vi "DeleteUser.vi"(3 "error in (no error)":errorcluster, 4 "User_Name":string, 5 "ID":string) -> (0 "error out":errorcluster)   [LabVIEW 2020]
uses:
  <vilib>/Utility/error.llb/DialogType.ctl
  Global1.vi
  <vilib>/addons/database/Connection.llb/DB Tools Open Connec (String).vi
  <vilib>/addons/database/Connection.llb/Conn Execute.vi
  <vilib>/addons/database/Recordset.llb/Rec Destroy - Connection.vi
  <vilib>/addons/database/NI_Database_API.lvlib
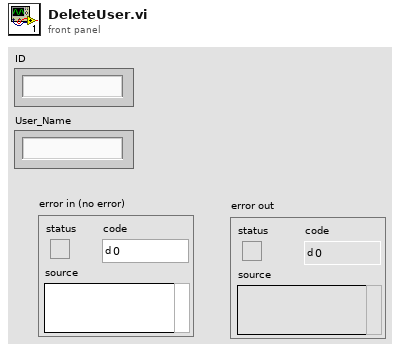
[diagram p1: front panel]
types:
  T1 = typedef "DialogType.ctl" = u16
  T2 = typedef "NI_Database_API.lvlib/Conn ObjectReference.ctl" = refnum<k1>
  T3 = typedef "NI_Database_API.lvlib/Rec ObjectReference.ctl" = refnum<k1>
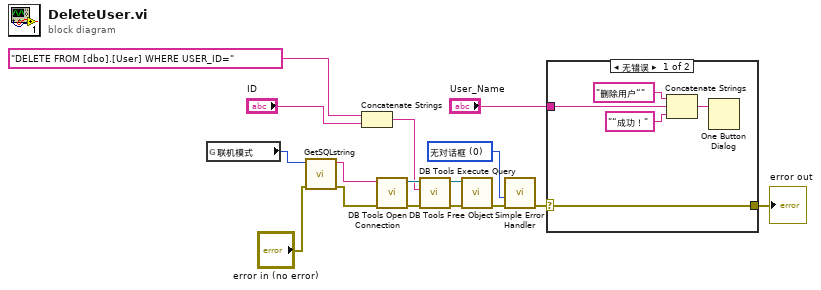
[diagram p0: block diagram]
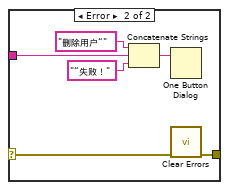
[diagram p2: hidden frame]
diagram:
  w11 = T1 0 items=["无对话框", "确定信息", "继续或停止信息", "确定信息＋警告", "继续/停止+警告"] ("type of dialog (OK msg:1)")
  n1 = global read "Global1.vi" "联机模式"() -> (w4:enum16{"单机", "联网"})
  n2 = call "GetSQLstring.vi"("错误输入"="error in (no error)", "联机模式"=w4) -> ("错误输出"=w1:errorcluster, "连接字符串"=w3:string)  [unwired: 8 in]
  n3 = Concatenate Strings("DELETE FROM [dbo].[User] WHERE USER_ID=", "ID") -> (w9:string)
  n4 = call-poly <vilib>:"DB Tools Open Connection.vi"("error in (no error)"=w1, "connection information"=w3) -> ("error out"=w16:errorcluster, "connection reference"=w15:T2)  [unwired: 6 in]
  n5 = call-poly <vilib>:"DB Tools Execute Query.vi"("error in (no error)"=w16, "SQL query"=w9, "connection reference"=w15) -> ("error out"=w14:errorcluster, "recordset reference"=w13:T3)  [unwired: 5 in]
  n6 = call-poly <vilib>:"DB Tools Free Object.vi"("error in (no error)"=w14, "recordset reference"=w13) -> ("error out"=w12:errorcluster)  [unwired: 8 in, 1 out]
  n7 = call <vilib>:"Simple Error Handler.vi"("type of dialog (OK msg:1)"=w11, "error in (no error)"=w12) -> ("error out"=w6:errorcluster)  [unwired: 3 in, 4 out]
  n8 = case shown="无错误" w6 {
    selector: w6 -> [w17 w22]
    tunnel: "User_Name" -> [w18 w24]
    tunnel: [w17 w23] -> w7
    frame No Error {
      n9 = Concatenate Strings("删除用户“" ("消息"), w18, "“成功！" ("消息")) -> (w21:string)
      n10 = One Button Dialog(message=w21) -> ()  [unwired: 1 in, 1 out]
    }
    frame Error {
      n11 = Concatenate Strings("删除用户“" ("消息"), w24, "“失败！" ("消息")) -> (w27:string)
      n12 = One Button Dialog(message=w27) -> ()  [unwired: 1 in, 1 out]
      n13 = call <vilib>:"Clear Errors.vi"("error in (no error)"=w22) -> ("error out"=w23:errorcluster)  [unwired: 5 in, 1 out]
    }
  }
  "error out" <- w7
